vi "Find Signal Period.vi"(6 "Measured Fs":dbl, 7 "X":dbl[](array[numeric])) -> (2 "Measured Period":dbl, 3 "Peaks Found":i32)   [LabVIEW 2014]
uses:
  <vilib>/Analysis/2dsp.llb/1D Auto Correlation (DBL).vi
  <vilib>/Analysis/baseanly.llb/Mean (DBL).vi
  <vilib>/Analysis/NI_AALPro.lvlib
  <vilib>/Analysis/NI_AAL_SigProc.lvlib
  <vilib>/Analysis/NI_AALBase.lvlib
panel:
  out "Mean Peak Diff":dbl format="%0.2f"
  out "X Signal Graph":dbl[](graph)
  out "AutoCorrelation Graph":cluster{"Locations":dbl[], "Amplitudes":dbl[]}[](graph)
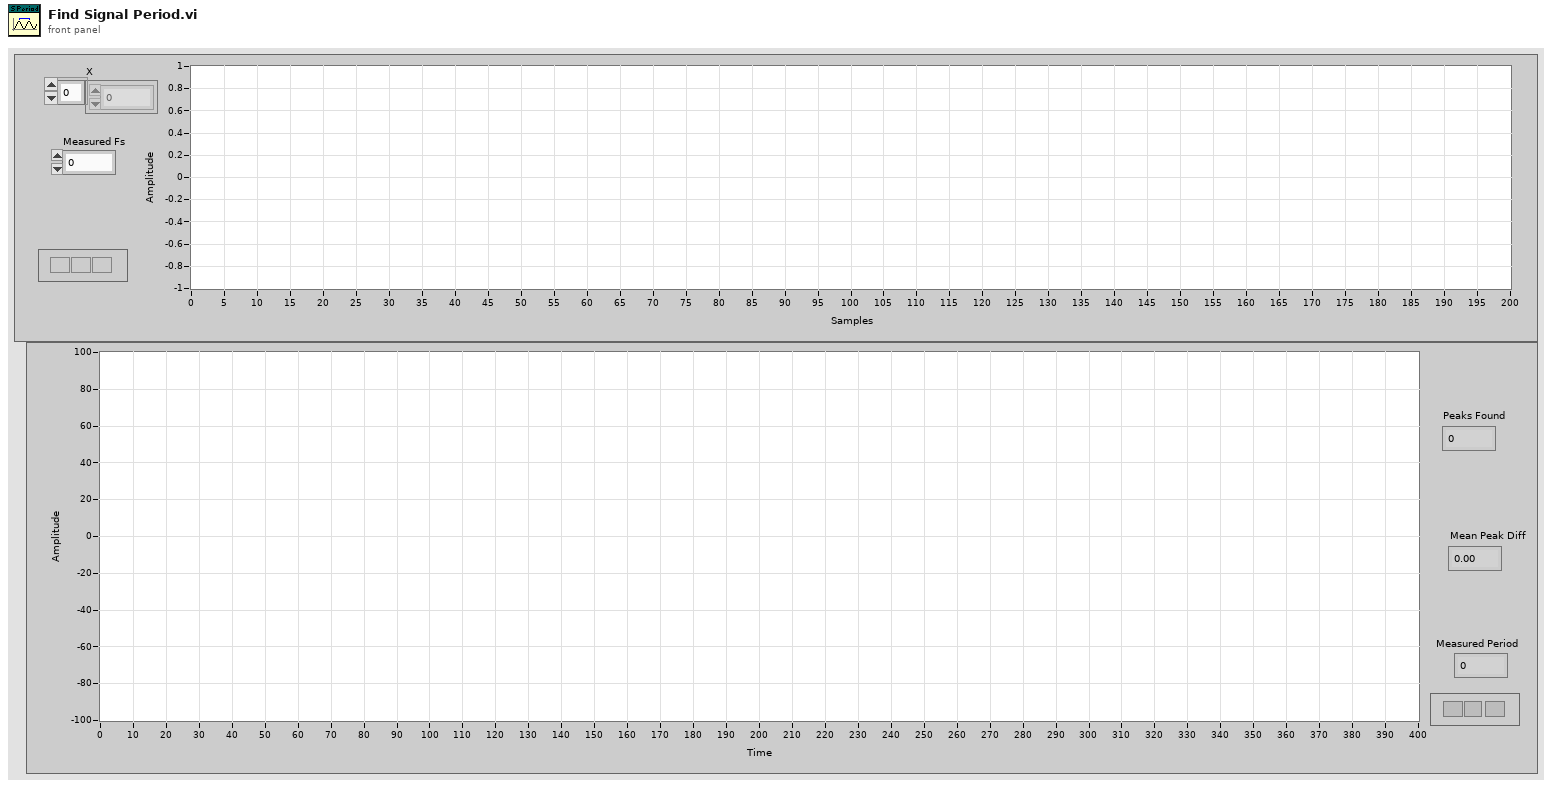
[diagram p1: front panel]
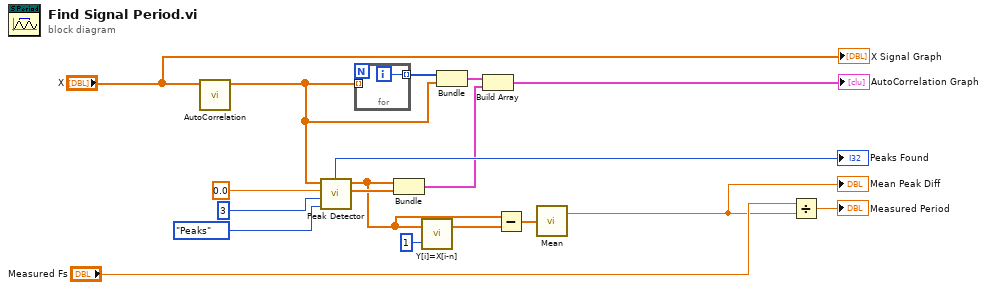
[diagram p0: block diagram]
diagram:
  n1 = call-poly <vilib>:"AutoCorrelation.vi"("X"="X") -> ("Rxx"=w12:dbl[])  [unwired: 9 in, 1 out]
  n2 = call <vilib>:"Peak Detector.vi"("peaks/valleys"=enum32{"Peaks", "Valleys"}."Peaks", "width"=3, "threshold"=0.0, "X"=w12) -> ("Amplitudes"=w6:dbl[], "Locations"=w1:dbl[], "# found"=→"Peaks Found":i32)  [unwired: 3 in, 2 out]
  n3 = for {
    tunnel: w12 -> [_] mode=indexing
    tunnel: [w19] -> w13 mode=indexing
    i -> [w19]
  }
  n4 = Bundle("Locations"=w1, "Amplitudes"=w6) -> (w10:cluster{"Locations":dbl[], "Amplitudes":dbl[]})  [unwired: 1 in]
  n5 = call <vilib>:"Y[i]=X[i-n].vi"("shifts: n"=1, "Input Array"=w1) -> ("Shifted Array"=w5:dbl[])  [unwired: 1 out]
  n6 = Bundle(w13, "Rxx"=w12) -> (w11:cluster{i32[], "Rxx":dbl[]})  [unwired: 1 in]
  n7 = Build Array(w11, w10) -> (→"AutoCorrelation Graph":cluster{"Locations":dbl[], "Amplitudes":dbl[]}[])
  n8 = Subtract(x=w1, y=w5) -> (x-y=w7:dbl[])
  n9 = call-poly <vilib>:"Mean.vi"("X"=w7) -> ("mean"=w3:dbl)  [unwired: 1 out]
  "Mean Peak Diff" <- w3
  n10 = Divide(x="Measured Fs", y=w3) -> (x/y=→"Measured Period":dbl)
  "X Signal Graph" <- "X"
